vi "VI_QUBE_collect_data.vi"() -> ()   [LabVIEW 2021]
uses:
  <vilib>/Simulation/Scripting/Companion Diagram/SimConfigNode/SimParams.ctl
  <vilib>/Simulation/Scripting/Companion Diagram/SimConfigNode/_simSolvers.ctl
  <vilib>/Simulation/Implementation/Shared/SIMSCR Execution Mode.ctl
  <vilib>/Platform/TimedLoop/XDataNode/timing_clust.ctl
  <vilib>/Platform/TimedLoop/XDataNode/nitl_modes.ctl
  <vilib>/Platform/TimedLoop/XDataNode/wakeup.ctl
  <vilib>/Simulation/Param Hierarchy/Typedefs/SIMPH Param Control Actions.ctl
  <vilib>/Simulation/Implementation/Shared/NILVSim_ParamChanged.vi
  <vilib>/Simulation/Implementation/Shared/NILVSim_FinishedLate.vi
  <vilib>/Simulation/Implementation/Shared/NILVSIM_BeginStep.vi
  <vilib>/Analysis/baseanly.llb/A x B.vi
  <vilib>/Analysis/baseanly.llb/Real A x B.vi
  <vilib>/Simulation/SignalArithmetic/Implementation/NILVSim Gain.llb/SIM Gain (scalar).vi
  <vilib>/Simulation/SignalDisplay/Implementation/NILVSim Time Waveform.llb/SIM Time Waveform (scalar).vi
  <vilib>/Simulation/ContinuousLinear/Implementation/NILVSim Transfer Function Direct.llb/SIM Transfer Function Direct (SISO).vi
  <vilib>/Simulation/Utility/Implementation/SIM Time.vi
  <vilib>/Simulation/Utility/Implementation/SIM Halt.vi
  <vilib>/Simulation/DataSources/Implementation/NILVSim Signal Generator.llb/SIM Signal Generator (scalar).vi
  <vilib>/Simulation/Implementation/Shared/SIM Is Init or Final Stage.vi
  <vilib>/Simulation/Implementation/Shared/NILVSim_Manager.vi
  <vilib>/Utility/error.llb/Clear Errors.vi
  <vilib>/Simulation/Implementation/Shared/NILVSim_FinalizeModel.vi
  <vilib>/Simulation/Implementation/Shared/SIM Unbundle Sim Info.vi
  <vilib>/Simulation/Implementation/Shared/SIMSH Read Queue.vi
  <vilib>/Simulation/Implementation/Shared/NILVSim_Initialize.vi
  <vilib>/Analysis/Matrix/Numeric/Conversions/Matrix To Array.vi
  <vilib>/Analysis/Matrix/Numeric/Conversions/Matrix To Array - RM.vi
  <vilib>/Simulation/Utility/Implementation/NILVSim Get Time and IsAcceptedStep.vi
  <vilib>/Simulation/Implementation/Shared/NILVSim_GetModelError.vi
  <vilib>/Simulation/Implementation/Shared/SIM Bundle Sim Info.vi
  <vilib>/Simulation/Scripting/Companion Diagram/SimConfigNode/SimDog.xnode
  <vilib>/Quanser/Rapid Control Prototyping Toolkit/hardware/HIL Immediate IO/_TypeSpecific/CL HIL Read Encoder (Vector).vi
  <vilib>/Quanser/Rapid Control Prototyping Toolkit/hardware/HIL Immediate IO/CL HIL Read.vi
  <vilib>/Quanser/Rapid Control Prototyping Toolkit/hardware/HIL Immediate IO/_TypeSpecific/CL HIL Write Analog (Scalar).vi
  <vilib>/Quanser/Rapid Control Prototyping Toolkit/hardware/HIL Immediate IO/CL HIL Write.vi
  <vilib>/Quanser/Rapid Control Prototyping Toolkit/hardware/HIL Board/HIL Board.lvclass
  <vilib>/Platform/TimedLoop/XDataNode/XDataNode.xnode
  <vilib>/Simulation/Implementation/XNodeFramework/SimXNode/SimX.xnode
  <vilib>/addons/System Identification/NI_SysID.lvlib
  <vilib>/Analysis/NI_AALBase.lvlib
  <vilib>/Analysis/Matrix/NI_Matrix.lvlib
  <vilib>/Platform/TimedLoop/XDataNode/XDNodeRunTimeDep.lvlib
  <vilib>/Simulation/Implementation/Shared/NI_SIM_Implementation.lvlib
panel:
  out "Iteration":i32
  out "Rotary arm speed q3 (rad/s)":waveform(dbl)(graph)
  out "Pendulum arm angle q2 (rad)":waveform(dbl)(graph)
  out "Pendulum arm speed q4 (rad/s)":waveform(dbl)(graph)
  out "Rotary arm angle q1 (rad)":waveform(dbl)(graph)
  in  "Timestep (s)":dbl
  in  "Control Duration (s)":dbl
  in  "Recording Duration (s)":dbl
  in  "Excitation Duration (s)":dbl
  out "Control input (V)":waveform(dbl)(graph)
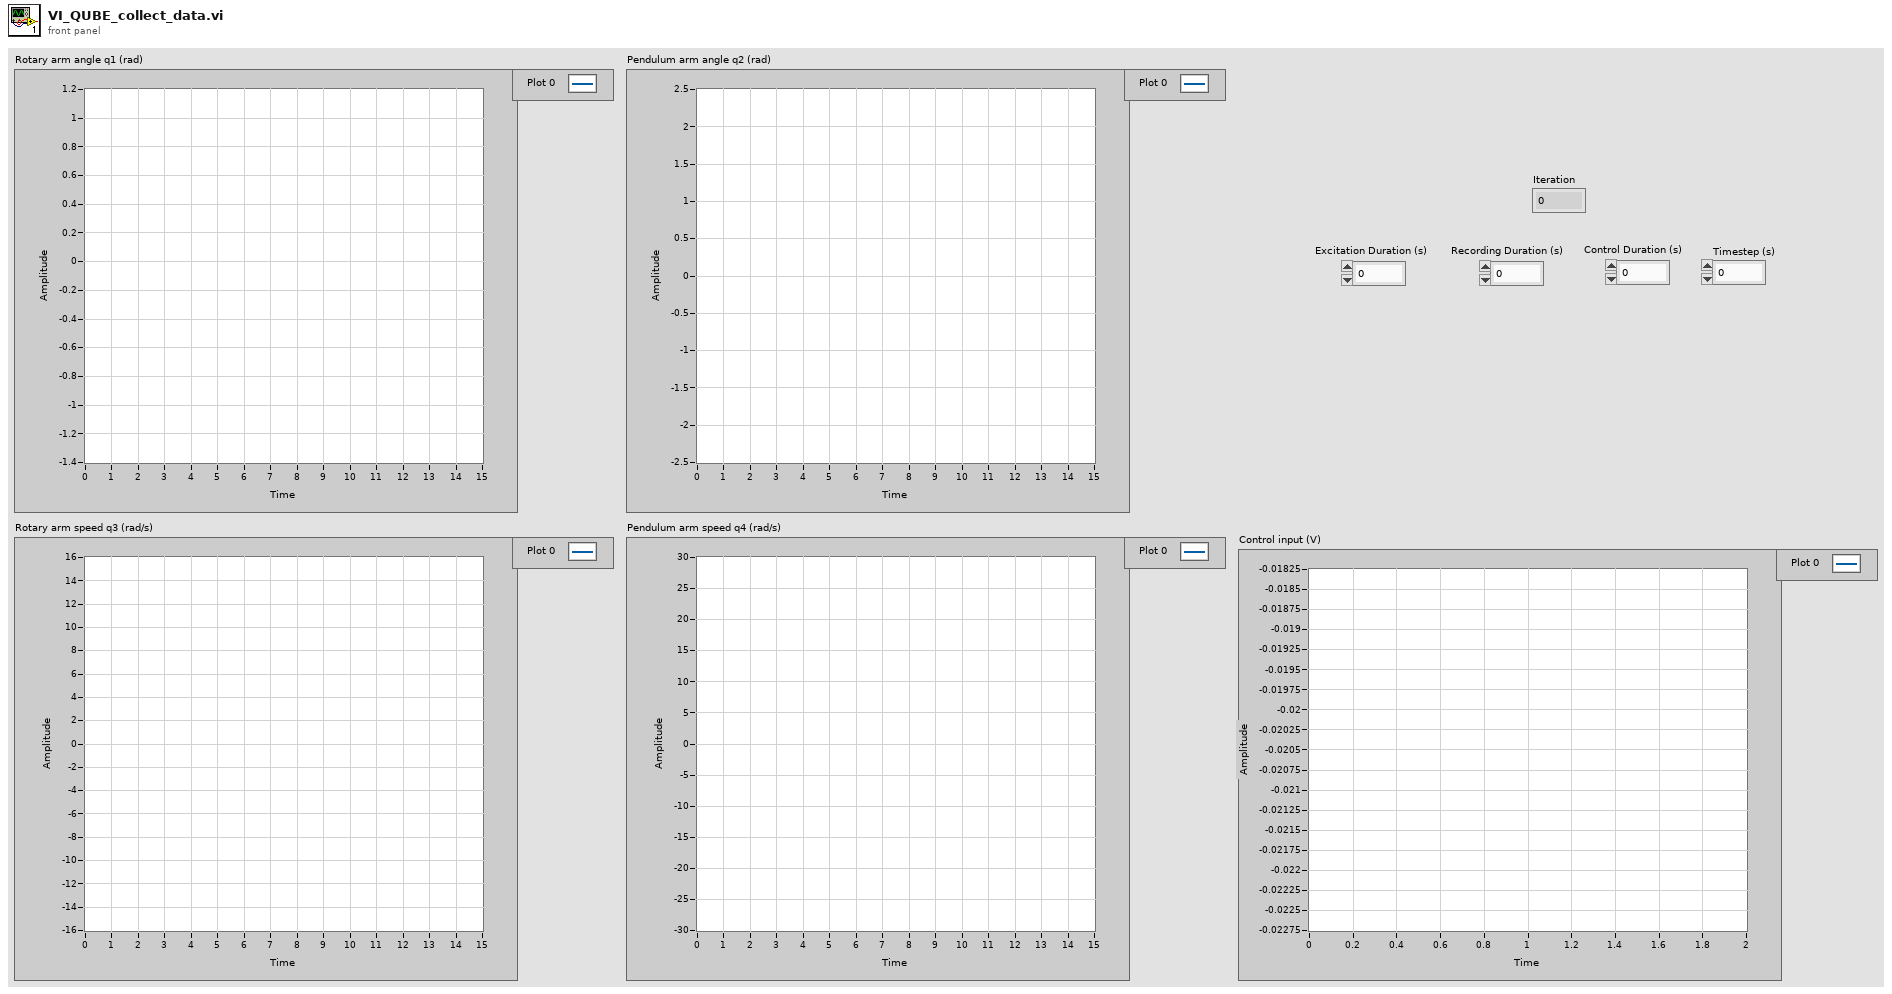
[diagram p1: front panel]
types:
  T1 = enum16{"open", "replace", "create", "open or create", "replace or create", "replace or create with confirmation"}
  T2 = typedef "SIMSCR Execution Mode.ctl" = enum16{"Simulate to Completion", "Single Time-Step Simulation (Fixed Step Only)"}
  T3 = typedef "XDNodeRunTimeDep.lvlib/timing_clust.ctl" = cluster{"Expected End [f-1]":u64, "Actual End [f-1]":u64, "Finished Late? [f-1]":bool, "Expected End [i-1]":u64, "Actual End [i-1]":u64, "Finished Late? [i-1]":bool, "Expected Start [i]":u64, "Actual Start [i]":u64, "Expected Start [f]":u64, "Actual Start [f]":u64, "Source Name":string, "Structure Name":string, "Period":i64, "Deadline":i64, "Offset":i64, "Start":i64, "Priority":i32, "Timeout":i32, "Mode":T4, "Wakeup Reason":T5, "Error":errorcluster, "Source Type":string, "Secondary Source Type":string, "Global End Time":u64, "Global Start Time":u64, "Frame Duration":u64, "Iteration Duration":u64, "Assigned CPU":i32, "I/O Scan Engine Mode":u32}
  T4 = typedef "XDNodeRunTimeDep.lvlib/nitl_modes.ctl" = enum32{"No Change", "Process missed periods, maintain original phase", "Discard missed periods, maintain original phase", "Process missed periods, ignore original phase", "Discard missed periods, ignore original phase"}
  T5 = typedef "XDNodeRunTimeDep.lvlib/wakeup.ctl" = enum32{"Normal", "Aborted", "Asynchronous wakeup", "Timing source error", "Timed loop error", "Timeout"}
  T6 = typedef "SIMPH Param Control Actions.ctl" = enum16{"get params", "set params"}
  T7 = cluster{"SIMSH Sim Time":dbl, "HIL Read Encoder.vi":cluster{"counts":i32[], "error out":errorcluster}}
  T8 = cluster{"SIMSH Sim Time":dbl, "HIL Write Analog.vi":cluster{"error out":errorcluster}, "CL HIL Write Termination States":cluster{"error out":errorcluster}, "CL HIL Write Termination States - SIMSH":cluster{"SIMSH Sim Time":dbl, "Property Node":cluster{"Properties:board handle":i64}, "quanser_emi_support.*:quanser_emi_support_main":cluster{"error out":errorcluster}, "cl_hil_write_termination_states.*:cl_hil_write_termination_states_main":cluster{"error out":errorcluster}, "CL HIL Write Termination States":cluster{"handle":dbl}, "Type Cast":cluster{"*(type *) &x":dbl}}}
  T9 = typedef "SimParams.ctl" = cluster{"Initial Time (s)":dbl, "Final Time (s)":dbl, "Step Size (s)":dbl, "ODE Solver":T10, "Minimum Step Size (s)":dbl, "Maximum Step Size (s)":dbl, "Relative Tolerance":dbl, "Absolute Tolerance":dbl, "Software Timing":bool, "Initial Step Size (s)":dbl, "Automatic Fixed Step Size?":bool, "Automatic Discrete Step Size?":bool, "Discrete Step Size (s)":dbl, "Calculate using Time Step":bool, "Solver Wired?":bool, "Prev.Frm.Expected End":u64, "Prev.Frm.Actual End":u64, "Prev.Frm.Finished Late?":bool, "Prev.Iter.Expected End":u64, "Prev.Iter.Actual End":u64, "Prev.Iter.Finished Late?":bool, "Expected Iteration Start":u64, "Actual Iteration Start":u64, "Expected Frame Start":u64, "Actual Frame Start":u64, "Source Name":string, "Name":string, "Period":i64, "Deadline":i64, "Offset":i64, "Start":i64, "Priority":i32, "Timeout":i32, "Processor":i32, "Mode":enum32{"No Change", "Process missed periods, maintain original phase", "Discard missed periods, maintain original phase", "Process missed periods, ignore original phase", "Discard missed periods, ignore original phase"}, "Wakeup reason":enum32{"Normal", "Aborted", "Asynchronous wakeup", "Timing source error", "Timed loop error", "Timeout"}, "Error":errorcluster, "Source Type":string, "Secondary Source Type":string, "Global End Time":u64, "Global Start Time":u64, "Full Solver Reset":bool, "Execution Mode":T2, "Nan/Inf Check":bool, "Custom Solver Library":string, "Solver Is Variable":bool, "custom solver name":string, "Signal Collection Decimation":u32}
  T10 = typedef "_simSolvers.ctl" = enum16{"Runge-Kutta 1 (Euler)", "Runge-Kutta 2", "Runge-Kutta 3", "Runge-Kutta 4", "Runge-Kutta 23 (variable)", "Runge-Kutta 45 (variable)", "BDF (variable)", "Adams-Moulton (variable)", "Rosenbrock (variable)", "Discrete States Only", "SDIRK 4 (variable)", "Radau 5 (variable)", "Radau 9 (variable)", "Radau 13 (variable)", "Radau [Variable Order] (variable)", "Gear's Method (variable)", "Linearizer", "State Query", "Trim Eval", "Custom Solver"}
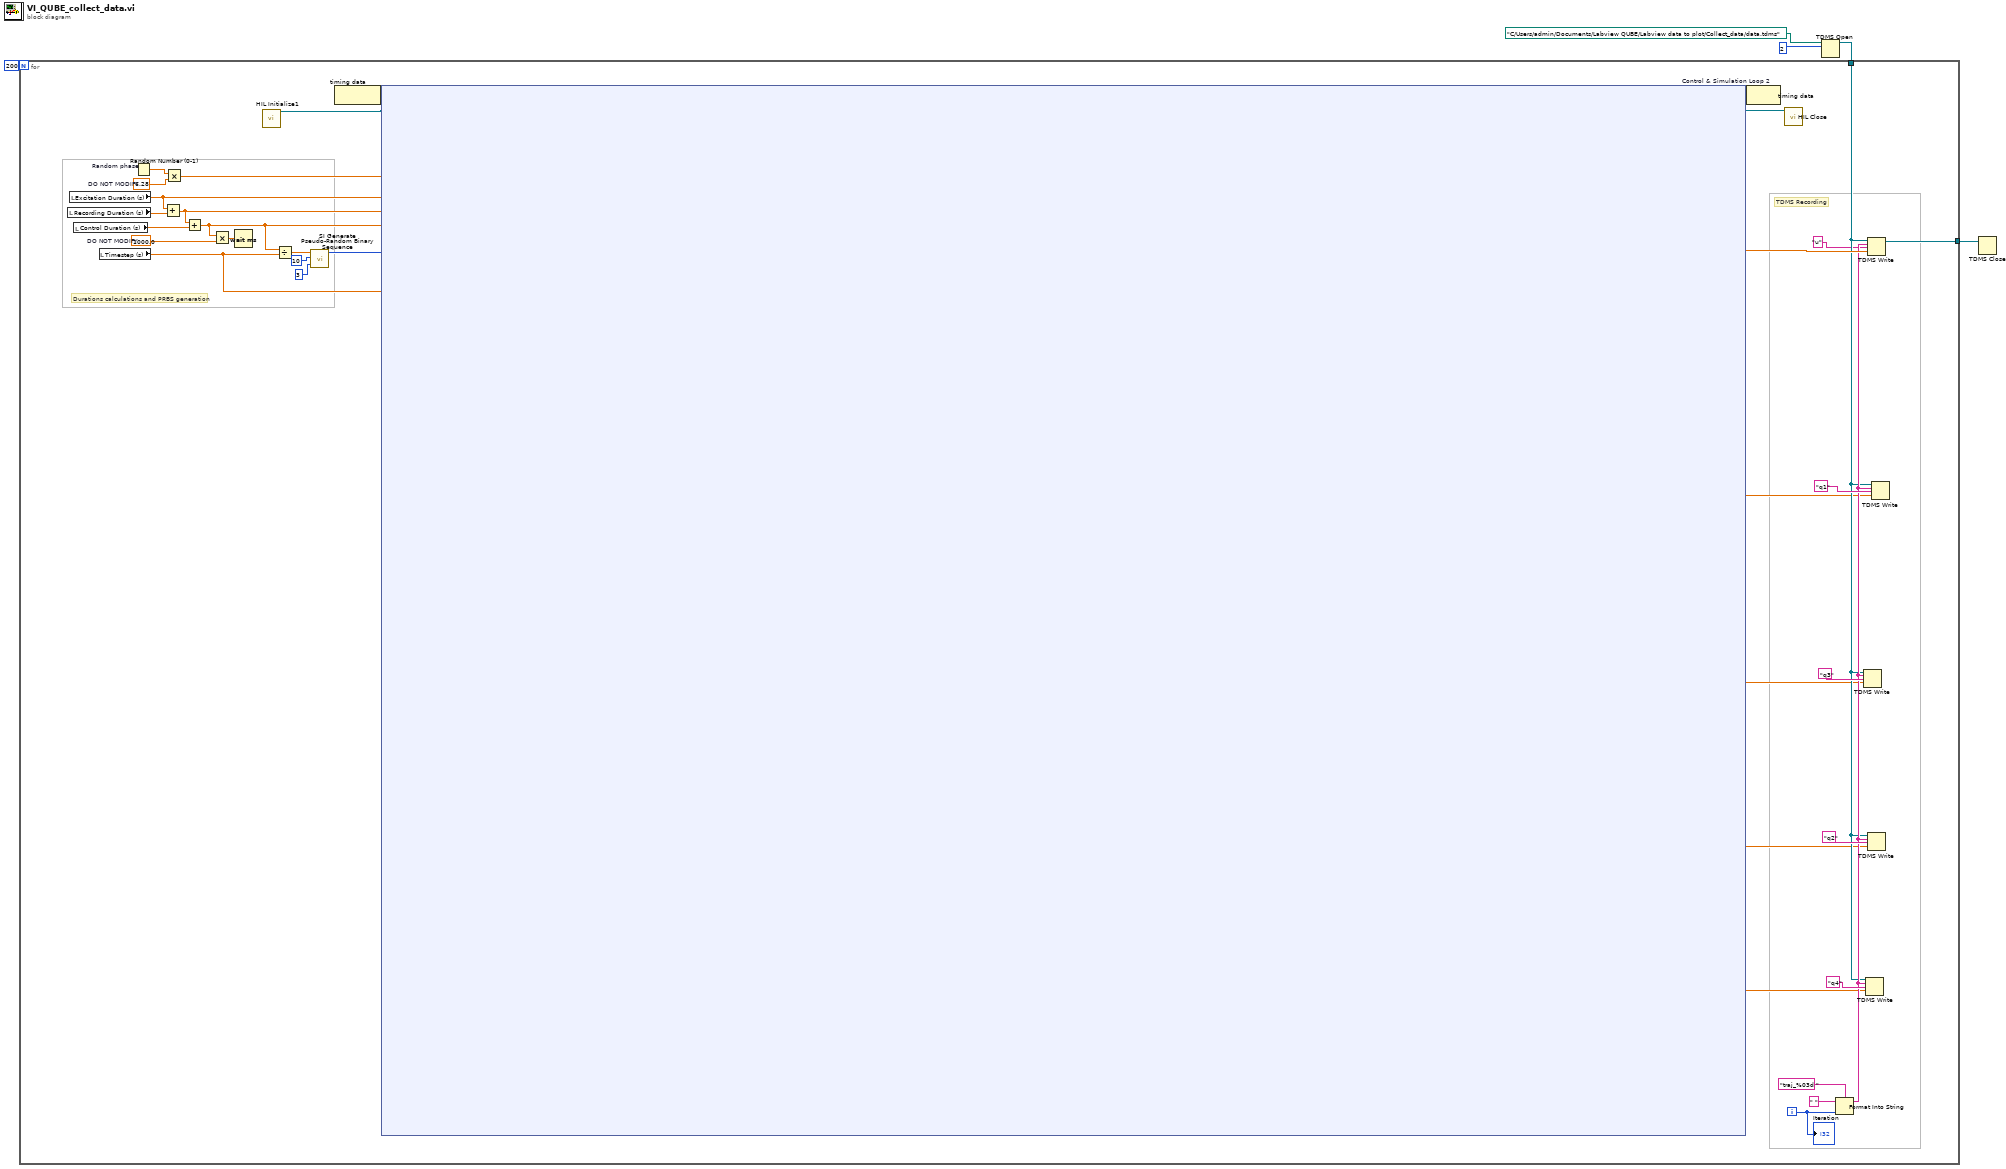
[diagram p0: block diagram]
diagram:
  n1 = TDMS Open(10:2 ("index 3"), 11:path "C:/Users/admin/Documents/Labview QUBE/Labview data to plot/Collect_data/data.tdms" ("file path (use dialog) 5")) -> (3:w4:refnum<k34>)  [unwired: 5 in, 1 out]
  n2 = for {
    N: 200 ("index") -> [_]
    tunnel: [w38] -> w5
    tunnel: w4 -> [w28]
    i -> [w35]
    w11 = 6.28  # DO NOT MODIFY
    w19 = 1000.0  # DO NOT MODIFY
    # "TDMS Recording"
    # "Durations calculations and PRBS generation"
    n3 = local read "Recording Duration (s)"() -> (w23:dbl)
    n4 = local read "Excitation Duration (s)"() -> (w24:dbl)
    n5 = local read "Control Duration (s)"() -> (w21:dbl)
    n6 = local read "Timestep (s)"() -> (w13:dbl)
    n7 = Random Number (0-1) "Random phase"() -> (number: 0 to 1=w12:dbl)
    n8 = Add(x=w24, y=w23) -> (x+y=w22:dbl)
    n9 = Multiply(x=w12, y=w11) -> (x*y=w10:dbl)
    n10 = Add(x=w22, y=w21) -> (x+y=w15:dbl)
    n11 = Multiply(x=w15, y=w19) -> (x*y=w20:dbl)
    n12 = Wait (ms)(milliseconds to wait=w20) -> ()  [unwired: 1 out]
    n13 = call "HIL Initialize1"() -> ("board out"=w26:refnum<class "HIL Board.lvclass">)  [unwired: 14 in, 1 out]
    n14 = Divide(x=w15, y=w13) -> (x/y=w18:dbl)
    n15 = call <vilib>:"SI Generate Pseudo-Random Binary Sequence.vi"("upsampling factor"=3 ("index"), "polynomial order"=10 ("index"), "samples"=w18) -> ("PRBS"=w14:u8[])  [unwired: 8 in]
    n16 = node-c288() -> (w40:variant)  [unwired: 1 in]
    n17 = node-c254 "Control & Simulation Loop 2"(w40, w26, w24, w22, w15, w14, w13, w10) -> (w39:variant, w37:dbl[], w25:refnum<class "HIL Board.lvclass">, w9:dbl[], w6:dbl[], w7:dbl[], w8:dbl[])
    n18 = node-c288(w39) -> ()  [unwired: 1 out]
    n19 = call <vilib>:"HIL Close.vi"("board in"=w25) -> ()  [unwired: 10 in, 1 out]
    n20 = Format Into String(format string="traj_%03d " ("initial string 3"), initial string=" " ("initial string 3"), w35) -> (resulting string=w29:string)  [unwired: 1 in, 1 out]
    n21 = TDMS Write(0:w28, 5:w29, 7:"q3", 9:w6) -> ()  [unwired: 2 in, 4 out]
    n22 = TDMS Write(0:w28, 5:w29, 7:"q4", 9:w8) -> ()  [unwired: 2 in, 4 out]
    n23 = TDMS Write(0:w28, 5:w29, 7:"u", 9:w37) -> (4:w38:refnum<k34>)  [unwired: 2 in, 3 out]
    n24 = TDMS Write(0:w28, 5:w29, 7:"q2", 9:w7) -> ()  [unwired: 2 in, 4 out]
    n25 = TDMS Write(0:w28, 5:w29, 7:"q1", 9:w9) -> ()  [unwired: 2 in, 4 out]
    "Iteration" <- w35
  }
  n26 = TDMS Close(11:w5) -> ()  [unwired: 1 in, 2 out]
